vi "sum.vi"() -> ()   [LabVIEW 2023]
panel:
  out "x+y":dbl
  in  "Y":dbl
  in  "X":dbl
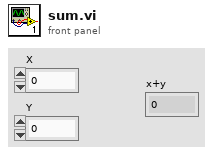
[diagram p1: front panel]
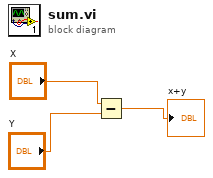
[diagram p0: block diagram]
diagram:
  n1 = Subtract(x="X", y="Y") -> (x-y=→"x+y":dbl)
